vi "macro_DrumSeq_Pulse.vi"   [LabVIEW 2019, in "Trajectory_Library.lvlib"]
uses:
  Trajectory_Library.lvlib
types:
  T1 = typedef "Trajectory_Library.lvlib/DrumSequence_Step_Enum.ctl" = enum16{"Do Nothing", "Step 1", "Step 2", "Step 3", "Step 4", "Step 5", "Step 6", "Step 7", "Step 8", "Step 9", "Step 10", "Step 11", "Step 12", "Step 13", "Step 14", "Step 15", "Step 16", "Step 17", "Step 18", "Step 19", "Step 20", "Step 21", "Step 22", "Step 23", "Step 24", "Step 25", "Step 26", "Step 27", "Step 28", "Step 29", "Step 30", "Step 31", "Step 32", "Cancel", "Initialize", "Error"}
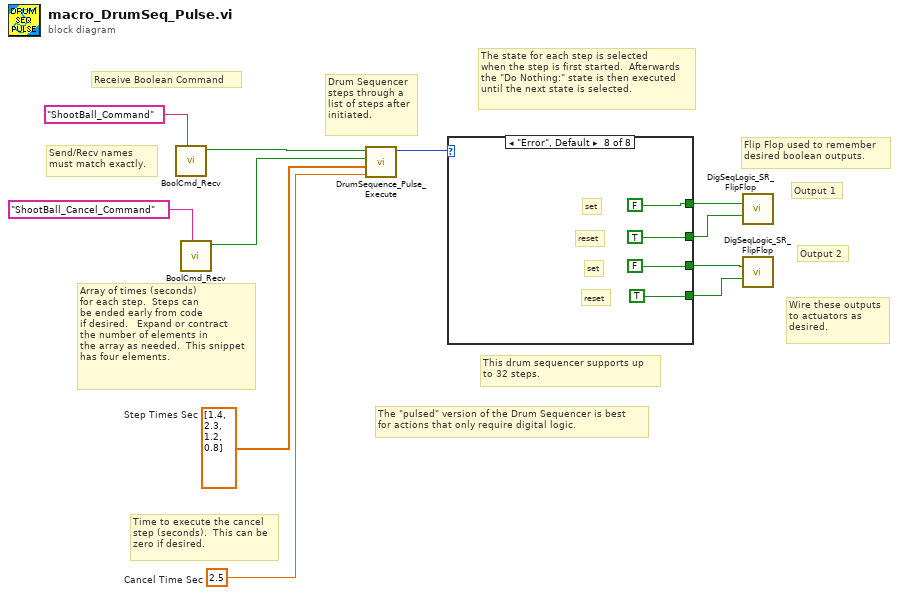
[diagram p0: block diagram]
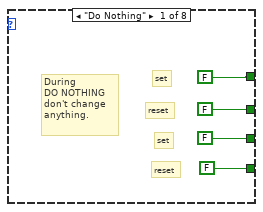
[diagram p2: hidden frame]
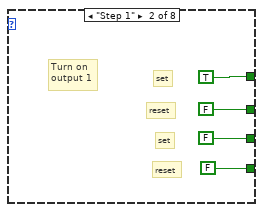
[diagram p3: hidden frame]
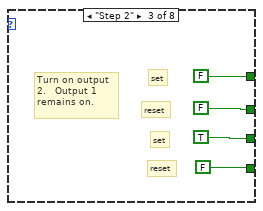
[diagram p4: hidden frame]
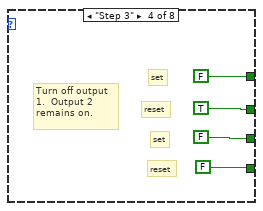
[diagram p5: hidden frame]
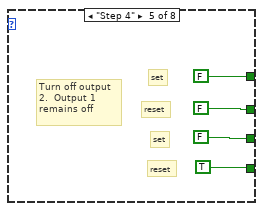
[diagram p6: hidden frame]
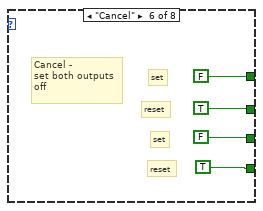
[diagram p7: hidden frame]
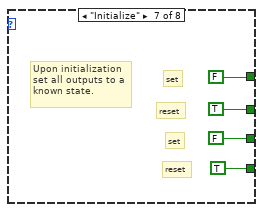
[diagram p8: hidden frame]
diagram:
  w6 = 2.5  # Cancel Time Sec
  w7 = dbl[] [1.4, 2.3, 1.2, 0.8]  # Step Times Sec
  # "This drum sequencer supports up\nto 32 steps."
  # "Wire these outputs\nto actuators as\ndesired."
  # "Output 2"
  # "Output 1"
  # "Flip Flop used to remember\ndesired boolean outputs."
  # "The \"pulsed\" version of the Drum Sequencer is best\nfor actions that only require digital logic."
  # "The state for each step is selected\nwhen the step is first started.  Afterwards\nthe \"Do Nothing:\" state is then executed\nuntil the next state is selected."
  # "Drum Sequencer\nsteps through a \nlist of steps after\ninitiated."
  # "Time to execute the cancel\nstep (seconds).  This can be\nzero if desired."
  # "Array of times (seconds)\nfor each step.  Steps can\nbe ended early from code\nif desired.   Expand or contract\nthe number of elements in\nthe array as needed.  This snippet\nhas four elements."
  # "Send/Recv names\nmust match exactly."
  # "Receive Boolean Command"
  n1 = call "BoolCmd_Recv.vi"("Command Name"="ShootBall_Command") -> ("New Request"=w10:bool)  [unwired: 9 in, 1 out]
  n2 = call "BoolCmd_Recv.vi"("Command Name"="ShootBall_Cancel_Command") -> ("New Request"=w8:bool)  [unwired: 9 in, 1 out]
  n3 = call "DrumSequence_Pulse_Execute.vi"("Cancel Time Sec"=w6, "Step Times Sec"=w7, "Cancel"=w8, "Initiate"=w10) -> ("Step Number State"=w5:T1)  [unwired: 4 in, 3 out]
  n4 = case shown="\"Error\", Default" w5 {
    tunnel: [FALSE TRUE FALSE FALSE FALSE FALSE FALSE FALSE] -> w4
    tunnel: [FALSE FALSE FALSE TRUE FALSE TRUE TRUE TRUE] -> w3
    tunnel: [FALSE FALSE TRUE FALSE FALSE FALSE FALSE FALSE] -> w2
    tunnel: [FALSE FALSE FALSE FALSE TRUE TRUE TRUE TRUE] -> w1
    frame "Do Nothing" {
      # "During \nDO NOTHING\ndon't change\nanything."
      # "reset"
      # "set"
      # "reset"
      # "set"
    }
    frame "Step 1" {
      # "Turn on \noutput 1"
      # "reset"
      # "set"
      # "reset"
      # "set"
    }
    frame "Step 2" {
      # "Turn on output\n2.   Output 1\nremains on."
      # "reset"
      # "set"
      # "reset"
      # "set"
    }
    frame "Step 3" {
      # "Turn off output\n1.  Output 2\nremains on."
      # "reset"
      # "set"
      # "reset"
      # "set"
    }
    frame "Step 4" {
      # "Turn off output\n2.  Output 1\nremains off"
      # "reset"
      # "set"
      # "reset"
      # "set"
    }
    frame "Cancel" {
      # "Cancel - \nset both outputs\noff"
      # "reset"
      # "set"
      # "reset"
      # "set"
    }
    frame "Initialize" {
      # "reset"
      # "set"
      # "reset"
      # "set"
      # "Upon initialization\nset all outputs to a\nknown state."
    }
    frame "Error", Default {
      # "reset"
      # "set"
      # "reset"
      # "set"
    }
  }
  n5 = call "DigSeqLogic_SR_FlipFlop.vi"("Set"=w4, "Reset"=w3) -> ()  [unwired: 12 in, 2 out]
  n6 = call "DigSeqLogic_SR_FlipFlop.vi"("Set"=w2, "Reset"=w1) -> ()  [unwired: 12 in, 2 out]
